vi "Pack for gRPC.vi"(8 "error in":errorcluster, 9 "configuration / results":enum16{"Configuration", "Results"}(ring), 10 "data value":variant, 11 "measurement customizations in":refnum<class "Measurement Plugin.lvclass">) -> (0 "error out":errorcluster, 2 "any":T1, 3 "measurement customizations out":refnum<class "Measurement Plugin.lvclass">)   [LabVIEW 2021, in "Ramp-Up Time_PMIC.lvlib" / "Measurement Plugin.lvclass"]
uses:
  Measurement Plugin.lvclass
  Measurement Plugin.lvclass/Measurement Plugin.ctl
  Measurement Configuration.ctl
  Ramp-Up Time_PMIC.lvlib
  Measurement Results.ctl
  a6012965-5700-4384-8228-972e71b6560c.vi
  2eca732d-dbaa-43bf-a7dd-ede2da65bc1b.vi
  <vilib>/Plug-In SDKs/Measurements/Measurement Plugin Service/Measurement Plugin Service.lvclass
  C:/Program Files/National Instruments/LabVIEW 2021/vi.lib/Plug-In SDKs/Measurements/Measurement Plugin Service/Measurement Plugin Service.lvclass
  C:/pmic-labview/source/measurements/ramp-up time/Ramp-Up Time_PMIC/Advanced/Measurement Plugin.lvclass
  <vilib>/gRPC/LabVIEW gRPC Library/Shared/Any.ctl
  <vilib>/gRPC/LabVIEW gRPC Library/grpc-lvsupport-release.lvlib
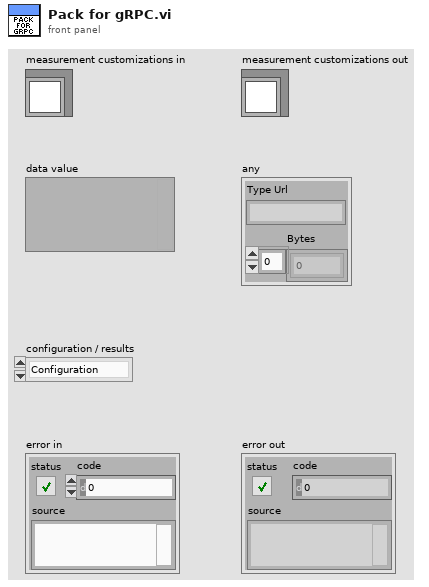
[diagram p1: front panel]
types:
  T1 = typedef "grpc-lvsupport-release.lvlib/Any.ctl" = cluster{"Type Url":string, "Bytes":u8[]}
  T2 = typedef "grpc-lvsupport-release.lvlib/grpcId.ctl" = u64
  T3 = typedef "Ramp-Up Time_PMIC.lvlib/Measurement Configuration.ctl" = cluster{"Source resource name":string, "Source current limit":dbl, "Source sample rate":dbl, "Source voltage set point 1":dbl, "Source voltage set point 2":dbl, "Source transient response":i32, "Source voltage gain bandwidth":dbl, "Source voltage compensation frequency":dbl, "Source voltage pole-zero ratio":dbl, "Source maximum power":dbl, "Source voltage ramp rate":dbl, "Source voltatge V2 time":dbl, "Source voltage V1 time":dbl, "Scope enable/disable":bool, "Scope output channel name":string, "Scope sample rate":dbl, "Scope probe attenuation":dbl, "Scope vertical range":dbl, "Scope vertical coupling":enum32{"AC", "DC"}}
  T4 = typedef "Ramp-Up Time_PMIC.lvlib/Measurement Results.ctl" = cluster{"Source voltage dt":dbl, "Source voltages":dbl[], "Scope amplitude dt":dbl, "Scope amplitudes":dbl[]}
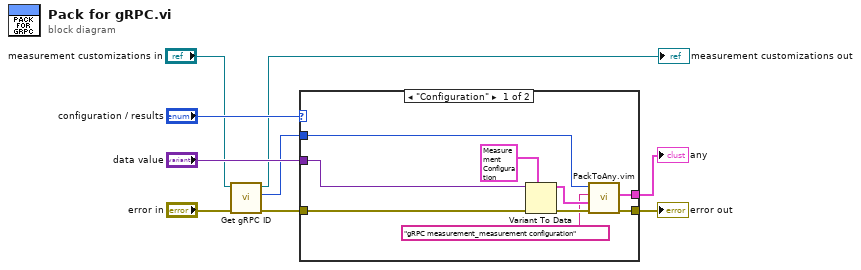
[diagram p0: block diagram]
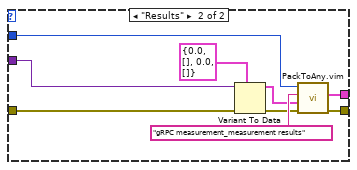
[diagram p2: hidden frame]
diagram:
  n1 = call <vilib>:"Get gRPC ID.vi"("error in"="error in", "measurement plugin service in"="measurement customizations in") -> ("error out"=w4:errorcluster, "gRPC ID"=w1:T2, "measurement plugin service out"=→"measurement customizations out":refnum<class "Measurement Plugin.lvclass">)  [unwired: 7 in]
  n2 = case shown="\"Configuration\"" "configuration / results" {
    tunnel: w4 -> [w18 w27]
    tunnel: "data value" -> [w17 w26]
    tunnel: w1 -> [w14 w22]
    tunnel: [w16 w24] -> w8
    tunnel: [w15 w23] -> w7
    frame "Configuration" {
      n3 = Variant To Data(error in=w18, type=T3 {"Source resource name"="Lorem ipsum dolor sit", "Source current limit"=1.2, "Source sample rate"=32.0, "Source voltage set point 1"=32.0, "Source voltage set point 2"=64.0, "Source transient response"=64, "Source voltage gain bandwidth"=-32.0, "Source voltage compensation frequency"=-32.0, "Source voltage pole-zero ratio"=-64.0, "Source maximum power"=-64.0, "Source voltage ramp rate"=1.0, "Source voltatge V2 time"=1.0, "Source voltage V1 time"=1.0, "Scope enable/disable"=TRUE, "Scope output channel name"="0", "Scope sample rate"=1800000.0, "Scope probe attenuation"=1.0, "Scope vertical range"=10.0, "Scope vertical coupling"=enum."DC"} ("measurement configuration"), Variant=w17) -> (data=w13:T3, error out=w12:errorcluster)
      n4 = call "PackToAny.vim"("error in"=w12, "Data To Pack"=w13, "Message Type"="gRPC measurement_measurement configuration", "gRPCid in"=w14) -> ("error out"=w16:errorcluster, "Any"=w15:T1)  [unwired: 5 in, 1 out]
    }
    frame "Results" {
      n5 = Variant To Data(error in=w27, type=T4 {"Source voltage dt"=0.0, "Source voltages"=[], "Scope amplitude dt"=0.0, "Scope amplitudes"=[]} ("Measurement Results"), Variant=w26) -> (data=w20:T4, error out=w19:errorcluster)
      n6 = call "PackToAny.vim"("error in"=w19, "Data To Pack"=w20, "Message Type"="gRPC measurement_measurement results", "gRPCid in"=w22) -> ("error out"=w24:errorcluster, "Any"=w23:T1)  [unwired: 5 in, 1 out]
    }
  }
  "error out" <- w8
  "any" <- w7
